vi "GUI Measurement setup.vi"(9 "FFmeter settings":T1={"AC Source"={"AC Source type"=enum."Fluke 5XXX calibrator", "VISA"="", "Ref. clock (Hz)"=0.0, "status ref"=refnum}, "TWM pipe"="\\\\.\\pipe\\TWM:server", "Measurement status ref"=refnum, "TWM Status ref"=refnum, "Abort ref"=refnum, "DC meter"={"DC meter type"=enum."H/A/K 3458", "DC meter VISA"="", "NPLC"=10, "status ref"=refnum}, "Measurement properties"={"Measurement frequencies (Hz)"=[1000.0], "Sampling frequency (Hz)"=500000.0, "Signal amplitude (V)"=4.5, "AC-DC settle time (s)"=20.0, "Record length (multiples of period)"=[1000.0, 10000.0, 1000.0], "Measurement template file"=path "", "Row of START keyword"=1, "Row of STOP keyword"=0, "Calculate RMS from samples"=FALSE, "AC-DC warm up time (s)"=300.0, "Measurement template line"=[], "DC meter readings No."=10}, "Skip waiting ref"=refnum, "Octave paths"={"GNU Octave path"=path "C:/Program Files/GNU Octave/Octave-6.2.0/mingw64/bin", "TWM+QWTB path"=path "C:/Users/labina/Desktop/TWM-1.8.7.0-full/octprog", "lvlib path"=path "D:/martin/WAC/WACsw - github/control_software/Filter function meter/external libraries/GOLPI 0.7.3.1 source distribution LV 20.0 32 bit/lv_proc.dll"}, "Template definition"={"Keywords column"=0, "Sig. freq. column"=1, "Rec. len. column"=2, "Meas. points. row min to read"=9, "Meas. points. row max to read"=1509, "Properties column"=4, "Properties row start"=1, "Properties row end"=5, "Keyword START regexp"="", "Keyword STOP regexp"=""}} {"Measurement properties"."Record length (multiples of period)" format="%#_3p"; "Measurement properties"."Sampling frequency (Hz)" format="%#_3p"; "Measurement properties"."Measurement frequencies (Hz)" format="%#_3p"}) -> (3 "FFmeter settings out":T1={"AC Source"={"AC Source type"=enum."Fluke 5XXX calibrator", "VISA"="", "Ref. clock (Hz)"=0.0, "status ref"=refnum}, "TWM pipe"="\\\\.\\pipe\\TWM:server", "Measurement status ref"=refnum, "TWM Status ref"=refnum, "Abort ref"=refnum, "DC meter"={"DC meter type"=enum."H/A/K 3458", "DC meter VISA"="", "NPLC"=10, "status ref"=refnum}, "Measurement properties"={"Measurement frequencies (Hz)"=[1000.0], "Sampling frequency (Hz)"=500000.0, "Signal amplitude (V)"=4.5, "AC-DC settle time (s)"=20.0, "Record length (multiples of period)"=[1000.0, 10000.0, 1000.0], "Measurement template file"=path "", "Row of START keyword"=1, "Row of STOP keyword"=0, "Calculate RMS from samples"=FALSE, "AC-DC warm up time (s)"=300.0, "Measurement template line"=[], "DC meter readings No."=10}, "Skip waiting ref"=refnum, "Octave paths"={"GNU Octave path"=path "C:/Program Files/GNU Octave/Octave-6.2.0/mingw64/bin", "TWM+QWTB path"=path "C:/Users/labina/Desktop/TWM-1.8.7.0-full/octprog", "lvlib path"=path "D:/martin/WAC/WACsw - github/control_software/Filter function meter/external libraries/GOLPI 0.7.3.1 source distribution LV 20.0 32 bit/lv_proc.dll"}, "Template definition"={"Keywords column"=0, "Sig. freq. column"=1, "Rec. len. column"=2, "Meas. points. row min to read"=9, "Meas. points. row max to read"=1509, "Properties column"=4, "Properties row start"=1, "Properties row end"=5, "Keyword START regexp"="", "Keyword STOP regexp"=""}} {"Measurement properties"."Record length (multiples of period)" format="%#_3p"; "Measurement properties"."Sampling frequency (Hz)" format="%#_3p"; "Measurement properties"."Measurement frequencies (Hz)" format="%#_3p"})   [LabVIEW 2020]
uses:
  Type definitions/FFmeter settings.ctl
  General AC source/Type definitions/AC Source.ctl
  General AC source/Type definitions/AC Source type.ctl
  General DC meter/Type definitions/DC meter.ctl
  General DC meter/Type definitions/DC meter type.ctl
  Measurement/Type definitions/Measuement properties.ctl
  Utilities/Type definitions/Template definition.ctl
  <vilib>/Utility/error.llb/Error Cluster From Error Code.vi
  <vilib>/ErrorRing/Error Ring.xnode
  external libraries/varilib/varilib.lvlib
panel:
  out "dc meter readings":i32=50000 caption="DC meter readings"
  in  "recalculate template":bool
  out "ac-dc warmup time":dbl=50000.0 caption="AC-DC settle time" format="%#_6p"
  out "Estimate as formatted text":string
  out "Meas points":i32=1 caption="Measurement points"
  in  "Calculate RMS\nfrom samples":bool
  out "ac-dc settle time":dbl=50000.0 caption="AC-DC settle time" format="%#_6p"
  out "Measurement freq. | Record length":dbl[][](array[numeric])=[[1000.0]]
  in  "load template":bool
  in  "Measurement template file":path
  in  "show connections":bool
  out "Signal amplitude (V)":dbl=1.0 caption="AC voltage amplitude"
  out "Sampling frequency (Hz)":dbl=50000.0 caption="Sampling frequency" format="%#_6p"
  out "gui_elements":refnum<vi>[](array[refnum])
  in  "save_and_quit":bool
  in  "cancel":bool
  # "Load the template and check loaded values here:"
  # "V"
  # "Hz"
  # "Who will make\nnice pictures?\n\nconnection setup here"
  # "s"
  # "s"
  # "Who will make\nnice pictures?\n\nwaveforms here"
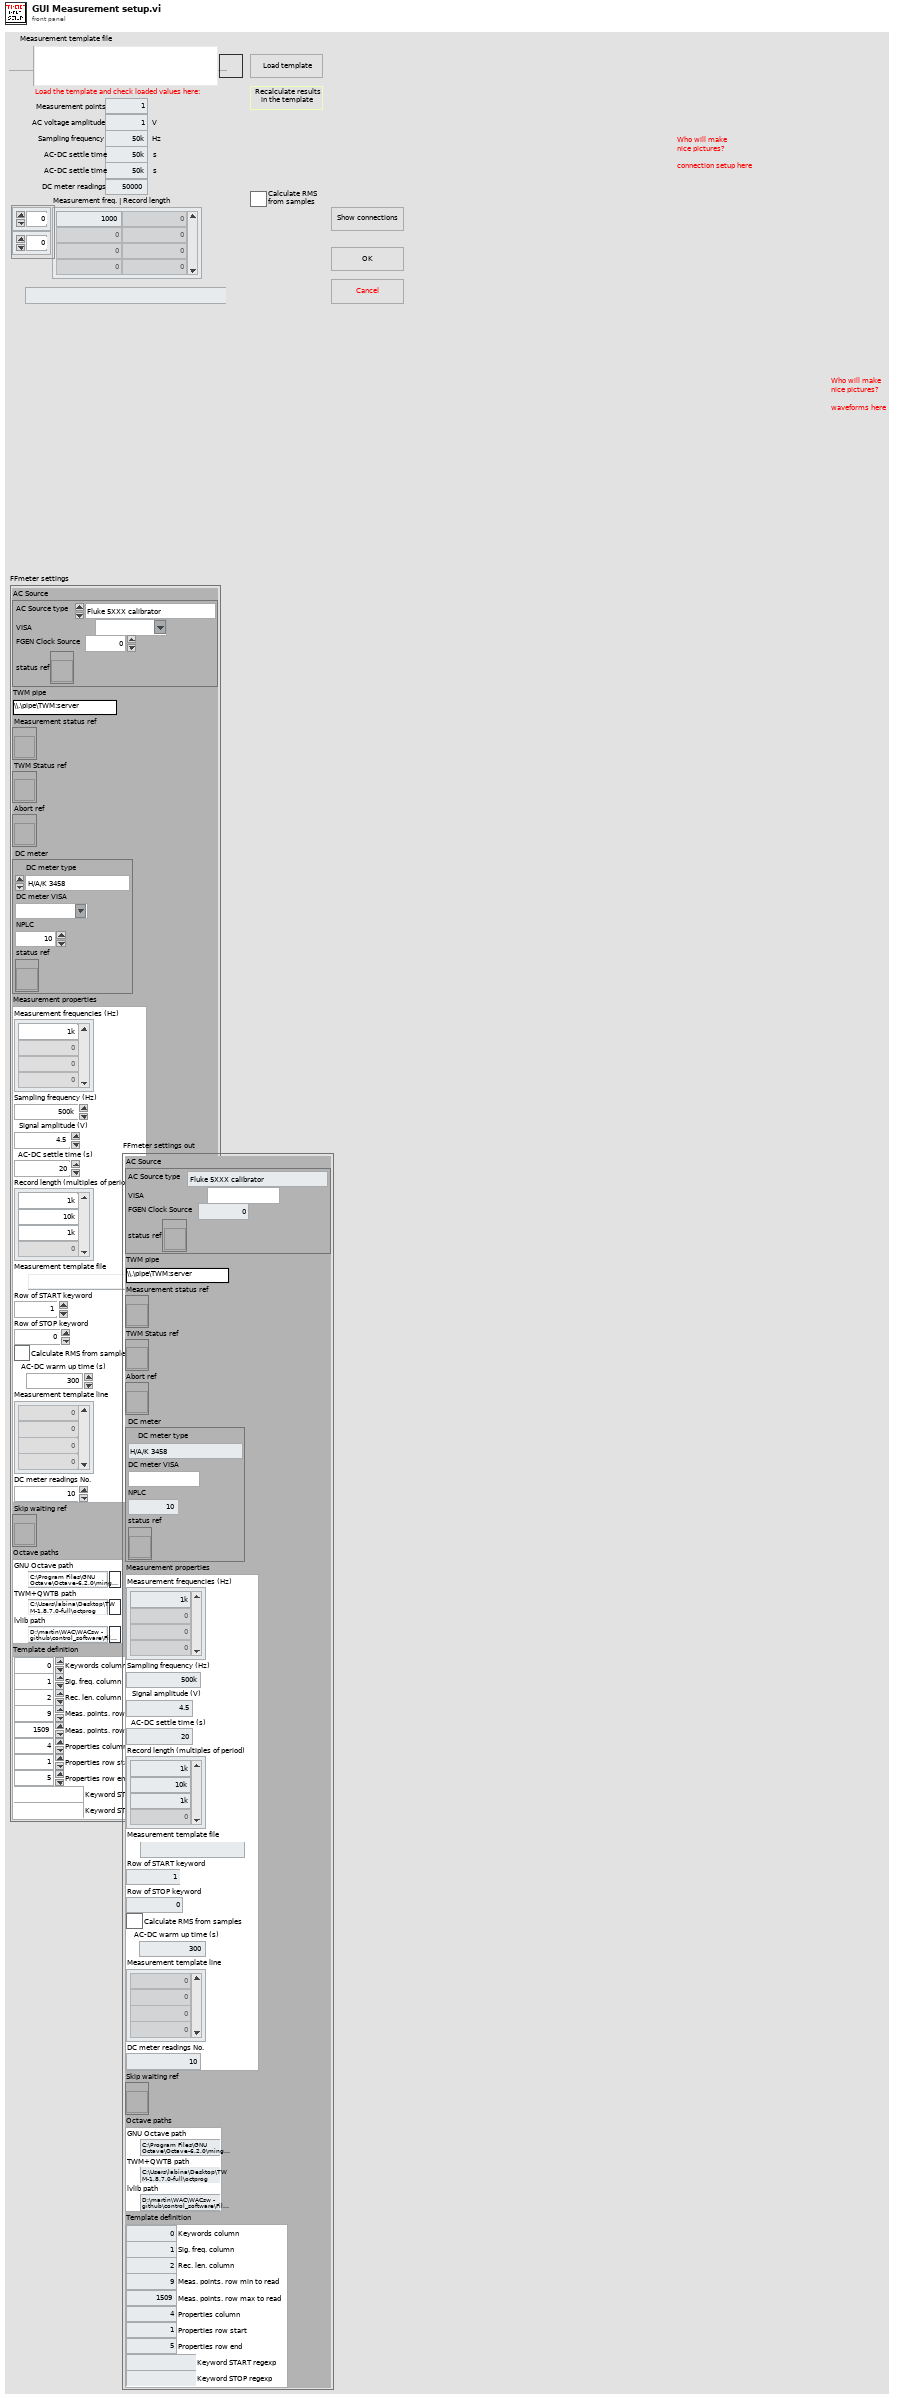
[diagram p1: front panel]
types:
  T1 = typedef "FFmeter settings.ctl" = cluster{"AC Source":T2, "TWM pipe":string, "Measurement status ref":refnum<vi>, "TWM Status ref":refnum<vi>, "Abort ref":refnum<vi>, "DC meter":T4, "Measurement properties":T6, "Skip waiting ref":refnum<vi>, "Octave paths":cluster{"GNU Octave path":path, "TWM+QWTB path":path, "lvlib path":path}, "Template definition":T7}
  T2 = typedef "AC Source.ctl" = cluster{"AC Source type":T3, "VISA":refnum<visa-resource-name>, "Ref. clock (Hz)":dbl, "status ref":refnum<vi>}
  T3 = typedef "AC Source type.ctl" = enum16{"Fluke 5XXX calibrator", "Tektronix AFG3101C", "dummy"}
  T4 = typedef "DC meter.ctl" = cluster{"DC meter type":T5, "DC meter VISA":refnum<visa-resource-name>, "NPLC":i32, "status ref":refnum<vi>}
  T5 = typedef "DC meter type.ctl" = enum16{"H/A/K 3458", "FLuke 8508A", "dummy"}
  T6 = typedef "Measuement properties.ctl" = cluster{"Measurement frequencies (Hz)":dbl[], "Sampling frequency (Hz)":dbl, "Signal amplitude (V)":dbl, "AC-DC settle time (s)":dbl, "Record length (multiples of period)":dbl[], "Measurement template file":path, "Row of START keyword":i32, "Row of STOP keyword":i32, "Calculate RMS from samples":bool, "AC-DC warm up time (s)":dbl, "Measurement template line":i32[], "DC meter readings No.":i32}
  T7 = typedef "Template definition.ctl" = cluster{"Keywords column":i32, "Sig. freq. column":i32, "Rec. len. column":i32, "Meas. points. row min to read":i32, "Meas. points. row max to read":i32, "Properties column":i32, "Properties row start":i32, "Properties row end":i32, "Keyword START regexp":string, "Keyword STOP regexp":string}
  T8 = enum32{"Bad", "Idle", "Run top level", "Running"}
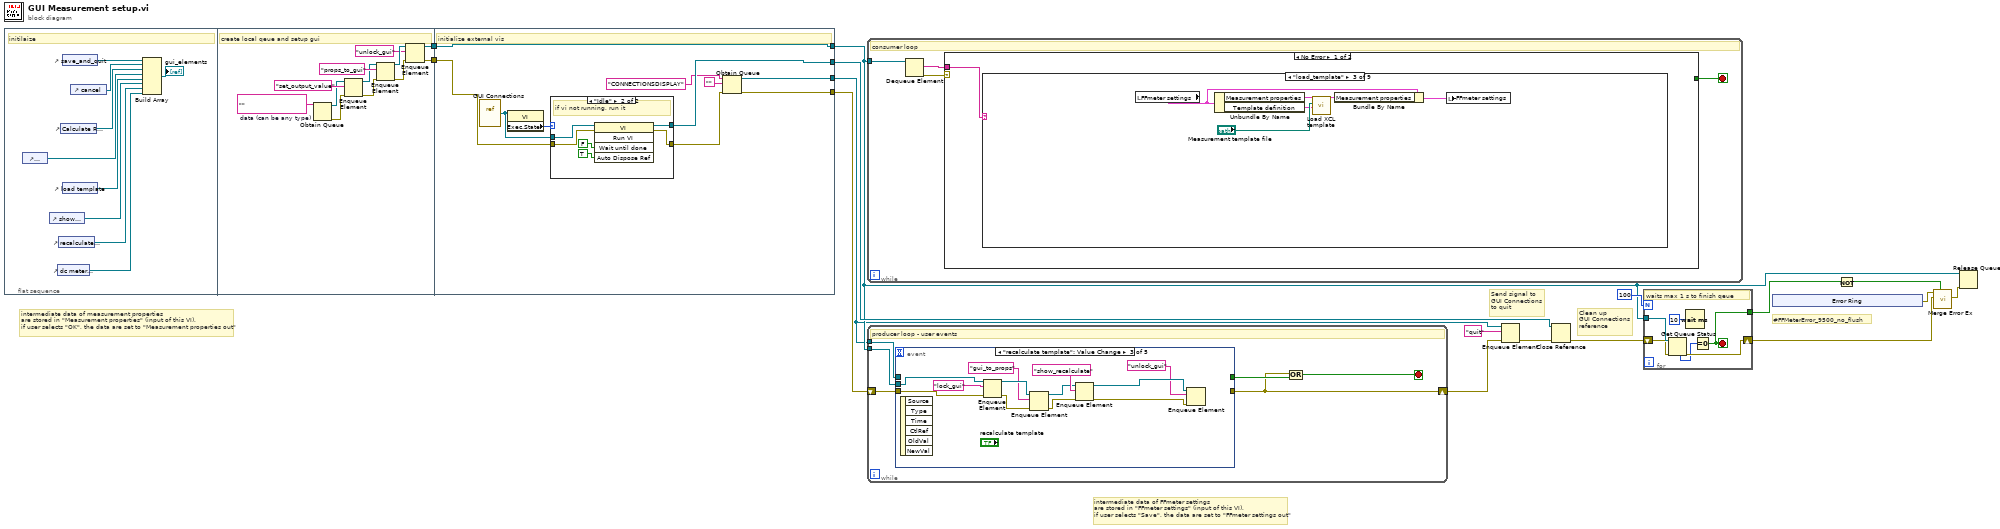
[diagram p0: block diagram]
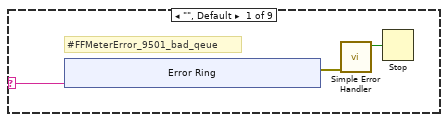
[diagram p3: hidden frame]
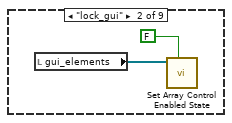
[diagram p4: hidden frame]
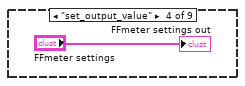
[diagram p5: hidden frame]
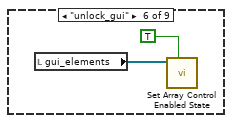
[diagram p7: hidden frame]
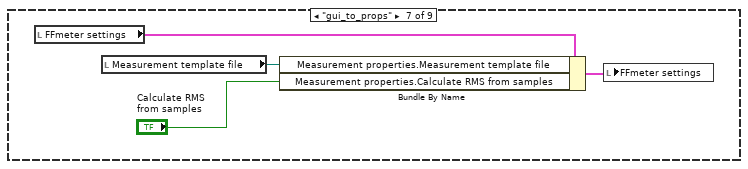
[diagram p8: hidden frame]
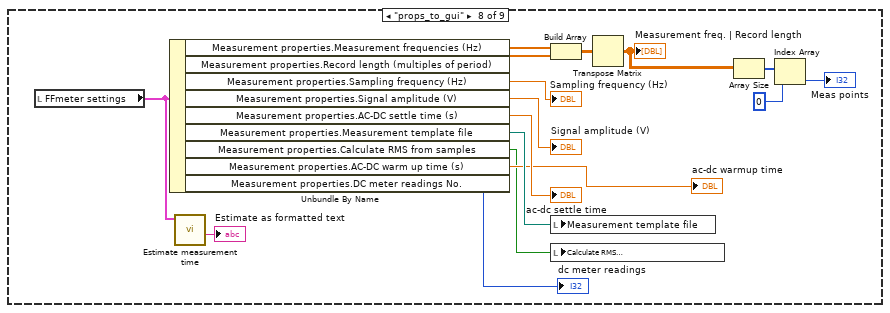
[diagram p9: hidden frame]
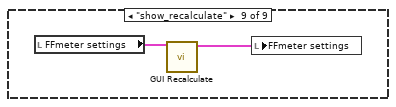
[diagram p10: hidden frame]
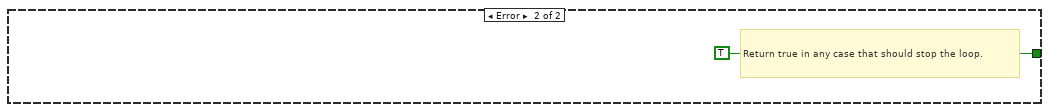
[diagram p11: hidden frame]
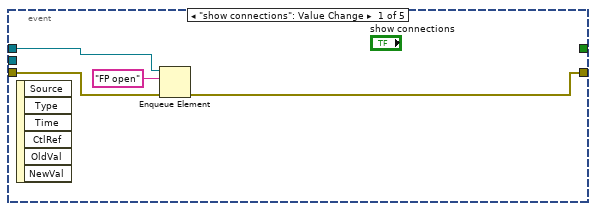
[diagram p12: hidden frame]
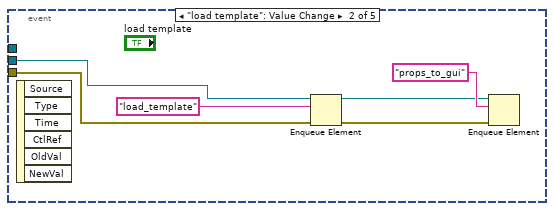
[diagram p13: hidden frame]
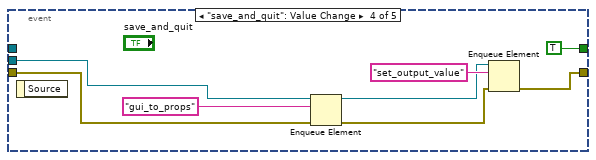
[diagram p14: hidden frame]
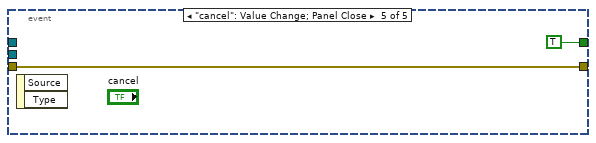
[diagram p15: hidden frame]
diagram:
  # "intermediate data of measurement properties\nare stored in \"Measurement properties\" (input of this VI),\nif user selects \"OK\", the data are set to \"Measurement properties out\""
  # "intermediate data of FFmeter settings\nare stored in \"FFmeter settings\" (input of this VI),\nif user selects \"Save\", the data are set to \"FFmeter settings out\""
  # "Send signal to\nGUI Connections\nto quit"
  # "Clean up\nGUI Connections\nreference"
  # "#FFMeterError_9500_no_flush"
  n1 = flat-sequence {
    tunnel: [w33] -> w9
    tunnel: [w34] -> w8
    tunnel: [w43] -> w10
    tunnel: [w47] -> w3
    tunnel: w9 -> [w47]
    tunnel: w8 -> [w46]
    tunnel: [w44] -> w2
    tunnel: [w45] -> w5
    frame #0 {
      # "initilaize"
      n2 = control-ref of="Measurement template file"() -> (w21:refnum<vi>)
      n3 = control-ref of="show connections"() -> (w19:refnum<vi>)
      n4 = control-ref of="dc meter readings"() -> (w17:refnum<vi>)
      n5 = control-ref of="recalculate template"() -> (w18:refnum<vi>)
      n6 = control-ref of="Calculate RMS\nfrom samples"() -> (w22:refnum<vi>)
      n7 = control-ref of="save_and_quit"() -> (w25:refnum<vi>)
      n8 = control-ref of="load template"() -> (w20:refnum<vi>)
      n9 = control-ref of="cancel"() -> (w24:refnum<vi>)
      n10 = Build Array(w25, w24, w22, w21, w20, w19, w18, w17) -> (→"gui_elements":refnum<vi>[])
    }
    frame #1 {
      w36 = ""  # data (can be any type)
      # "create local qeue and setup gui"
      n11 = Obtain Queue(element data type=w36) -> (queue out=w27:refnum<queue>, error out=w26:errorcluster)  [unwired: 4 in, 1 out]
      n12 = Enqueue Element(queue=w27, element="set_output_value", error in (no error)=w26) -> (queue out=w29:refnum<queue>, error out=w28:errorcluster)  [unwired: 1 in, 1 out]
      n13 = Enqueue Element(queue=w29, element="props_to_gui", error in (no error)=w28) -> (queue out=w32:refnum<queue>, error out=w35:errorcluster)  [unwired: 1 in, 1 out]
      n14 = Enqueue Element(queue=w32, element="unlock_gui", error in (no error)=w35) -> (queue out=w33:refnum<queue>, error out=w34:errorcluster)  [unwired: 1 in, 1 out]
    }
    frame #2 {
      # "initialize external vis"
      n15 = vi-ref "GUI Connections.vi"() -> (w41:refnum<vi>)
      n16 = property class="VI"(reference=w41) -> ("Exec.State"=w42:T8)  [unwired: 1 in, 2 out]
      n17 = case shown="\"Idle\"" w42 {
        tunnel: [w48 w55] -> w38
        tunnel: w46 -> [w48 w52]
        tunnel: [w49 w51] -> w45
        tunnel: w41 -> [w49 w50]
        frame "Bad", Default {
        }
        frame "Idle" {
          # "if vi not running, run it"
          n18 = invoke class="VI" method="Run VI"(reference=w50, error in=w52, "Wait until done"=FALSE ("Wait Until Done"), "Auto Dispose Ref"=TRUE ("Wait Until Done")) -> (reference out=w51:refnum<vi>, error out=w55:errorcluster)  [unwired: 1 in, 3 out]
        }
      }
      n19 = Obtain Queue(name (unnamed)="CONNECTIONSDISPLAY", element data type="", error in (no error)=w38) -> (queue out=w44:refnum<queue>, error out=w43:errorcluster)  [unwired: 2 in, 1 out]
    }
  }
  n20 = while {
    tunnel: w3 -> [w59]
    stop <- w56 stop-if-true
    # "consumer loop"
    n21 = Dequeue Element(queue=w59) -> (element=w57:string, error out=w58:errorcluster)  [unwired: 2 in, 2 out]
    n22 = case shown="No Error" w58 {
      tunnel: w57 -> [w60 _]
      tunnel: [_ TRUE] -> w56
      frame No Error {
        n23 = case shown="\"load_template\"" w60 {
          selector: w60 -> [w61 _ _ _ _ _ _ _ _]
          frame "", Default {
            # "#FFMeterError_9501_bad_qeue"
            n24 = xnode "Error Ring"("parameter 0"=w61) -> ("error out"=w63:errorcluster)
            n25 = call <vilib>:"Simple Error Handler.vi"("error in (no error)"=w63) -> ("error?"=w62:bool)  [unwired: 4 in, 4 out]
            n26 = Stop(stop? (T)=w62) -> ()
          }
          frame "lock_gui" {
            n27 = local read "gui_elements"() -> (w72:refnum<vi>[])
            n28 = call "Set Array Control Enabled State.vi"("enabled (T)"=FALSE, "reference array in"=w72) -> ()  [unwired: 8 in, 2 out]
          }
          frame "load_template" {
            n29 = local read "FFmeter settings"() -> (w76:T1)
            n30 = Unbundle By Name(w76) -> ("Measurement properties"=w75:T6, "Template definition"=w73:T7)
            n31 = call "Load XCL template.vi"("Template definition"=w73, "Measurement template file"="Measurement template file", "Measurement properties"=w75) -> ("Measurement properties out"=w74:T6)  [unwired: 8 in]
            n32 = Bundle By Name(cluster=w76, "Measurement properties"=w74) -> (w77:T1)
            n33 = local write "FFmeter settings"(w77) -> ()
          }
          frame "set_output_value" {
            "FFmeter settings out" <- "FFmeter settings"
          }
          frame "create_template" {
          }
          frame "unlock_gui" {
            n34 = local read "gui_elements"() -> (w81:refnum<vi>[])
            n35 = call "Set Array Control Enabled State.vi"("enabled (T)"=TRUE, "reference array in"=w81) -> ()  [unwired: 8 in, 2 out]
          }
          frame "gui_to_props" {
            n36 = local read "FFmeter settings"() -> (w84:T1)
            n37 = local read "Measurement template file"() -> (w82:path)
            n38 = Bundle By Name(cluster=w84, "Measurement properties.Measurement template file"=w82, "Measurement properties.Calculate RMS from samples"="Calculate RMS\nfrom samples") -> (w85:T1)
            n39 = local write "FFmeter settings"(w85) -> ()
          }
          frame "props_to_gui" {
            n40 = local read "FFmeter settings"() -> (w90:T1)
            n41 = Unbundle By Name(w90) -> ("Measurement properties.Measurement frequencies (Hz)"=w101:dbl[], "Measurement properties.Record length (multiples of period)"=w100:dbl[], "Measurement properties.Sampling frequency (Hz)"=→"Sampling frequency (Hz)":dbl, "Measurement properties.Signal amplitude (V)"=→"Signal amplitude (V)":dbl, "Measurement properties.AC-DC settle time (s)"=→"ac-dc settle time":dbl, "Measurement properties.Measurement template file"=w97:path, "Measurement properties.Calculate RMS from samples"=w86:bool, "Measurement properties.AC-DC warm up time (s)"=→"ac-dc warmup time":dbl, "Measurement properties.DC meter readings No."=→"dc meter readings":i32)
            n42 = call "Estimate measurement time.vi"("FFmeter settings"=w90) -> ("Estimate as formatted text"=→"Estimate as formatted text":string)  [unwired: 9 in, 1 out]
            n43 = Build Array(w101, w100) -> (w95:dbl[][])
            n44 = local write "Measurement template file"(w97) -> ()
            n45 = local write "Calculate RMS\nfrom samples"(w86) -> ()
            n46 = Transpose Matrix(1:w95) -> (0:w94:dbl[][])
            "Measurement freq. | Record length" <- w94
            n47 = Array Size(array=w94) -> (size(s)=w93:i32[])
            n48 = Index Array(array=w93, index=0) -> (element=→"Meas points":i32)
          }
          frame "show_recalculate" {
            n49 = local read "FFmeter settings"() -> (w103:T1)
            n50 = call "GUI Recalculate.vi"("FFmeter settings"=w103) -> ("FFmeter settings out"=w102:T1)  [unwired: 10 in]
            n51 = local write "FFmeter settings"(w102) -> ()
          }
        }
      }
      frame Error {
        # "Return true in any case that should stop the loop."
      }
    }
  }
  n52 = while {
    shift-right: [w106] -> w4
    shift-left: w10 -> [w109]
    tunnel: w3 -> [w110]
    tunnel: w2 -> [w105]
    stop <- w107 stop-if-true
    # "producer loop - user events"
    n53 = event shown="[2] \"recalculate template\": Value Change" {
      selector: _ -> [_ _ _ _ _]
      dyn-events: _ -> [_ _ _ _ _]
      timeout: _ -> [_ _ _ _ _]
      tunnel: w110 -> [_ w119 w127 w139 _]
      tunnel: w109 -> [w113 w118 w128 w138 w141]
      tunnel: [w112 _ _ w136 w141] -> w106
      tunnel: [_ _ _ TRUE ("cancel") TRUE ("cancel")] -> w108
      tunnel: w105 -> [w111 _ _ _ _]
      event "show connections": Value Change {
        n54 = event-data() -> ()  [unwired: 1 in, 6 out]
        n55 = Enqueue Element(queue=w111, element="FP open", error in (no error)=w113) -> (error out=w112:errorcluster)  [unwired: 1 in, 2 out]
      }
      event "load template": Value Change {
        n56 = event-data() -> ()  [unwired: 1 in, 6 out]
        n57 = Enqueue Element(queue=w119, element="load_template", error in (no error)=w118) -> (queue out=w115:refnum<queue>, error out=w117:errorcluster)  [unwired: 1 in, 1 out]
        n58 = Enqueue Element(queue=w115, element="props_to_gui", error in (no error)=w117) -> ()  [unwired: 1 in, 3 out]
      }
      event "recalculate template": Value Change {
        n59 = event-data() -> ()  [unwired: 1 in, 6 out]
        n60 = Enqueue Element(queue=w127, element="lock_gui", error in (no error)=w128) -> (queue out=w122:refnum<queue>, error out=w125:errorcluster)  [unwired: 1 in, 1 out]
        n61 = Enqueue Element(queue=w122, element="gui_to_props", error in (no error)=w125) -> (queue out=w123:refnum<queue>, error out=w124:errorcluster)  [unwired: 1 in, 1 out]
        n62 = Enqueue Element(queue=w123, element="show_recalculate", error in (no error)=w124) -> (queue out=w130:refnum<queue>, error out=w131:errorcluster)  [unwired: 1 in, 1 out]
        n63 = Enqueue Element(queue=w130, element="unlock_gui", error in (no error)=w131) -> ()  [unwired: 1 in, 3 out]
      }
      event "save_and_quit": Value Change {
        n64 = event-data() -> ()  [unwired: 1 in, 1 out]
        n65 = Enqueue Element(queue=w139, element="gui_to_props", error in (no error)=w138) -> (queue out=w133:refnum<queue>, error out=w137:errorcluster)  [unwired: 1 in, 1 out]
        n66 = Enqueue Element(queue=w133, element="set_output_value", error in (no error)=w137) -> (error out=w136:errorcluster)  [unwired: 1 in, 2 out]
      }
      event "cancel": Value Change; Panel Close {
        n67 = event-data() -> ()  [unwired: 1 in, 2 out]
      }
    }
    n68 = Or(x=w106, y=w108) -> (x .or. y?=w107:bool)
  }
  n69 = Enqueue Element(queue=w2, element="quit", error in (no error)=w4) -> (error out=w7:errorcluster)  [unwired: 1 in, 2 out]
  n70 = Close Reference(reference=w5, error in (no error)=w7) -> (error out=w1:errorcluster)
  n71 = for {
    N: 100 -> [_]
    tunnel: w3 -> [w148]
    shift-right: [w146] -> w13
    shift-left: w1 -> [w147]
    tunnel: [w143] -> w11
    stop <- w143 stop-if-true
    # "waits max 1 s to finish qeue"
    n72 = Get Queue Status(queue=w148, error in (no error)=w147) -> (error out=w146:errorcluster, # elements in queue=w144:i32)  [unwired: 1 in, 6 out]
    n73 = Wait (ms)(milliseconds to wait=u32 10) -> ()  [unwired: 1 out]
    n74 = Equal To 0?(x=w144) -> (x = 0?=w143:bool)
  }
  n75 = xnode "Error Ring"() -> ("error out"=w14:errorcluster)
  n76 = Not(x=w11) -> (.not. x?=w15:bool)
  n77 = call "Merge Error Ex.vi"("Is error? (False)"=w15, "main error in (no error)"=w13, "second error in"=w14) -> ("error out"=w12:errorcluster)  [unwired: 8 in]
  n78 = Release Queue(queue=w3, error in (no error)=w12) -> ()  [unwired: 1 in, 3 out]
